vi "Read Register.vi"(6 "Read Delay ms (5)":u32=5, 7 "SPI Peripheral":refnum<class "SPI Peripheral.lvclass">, 8 "error in (no error)":errorcluster, 9 "Len":u8, 10 "Register":u8 format="%.0x") -> (0 "error out":errorcluster, 1 "Data":string)   [LabVIEW 2020, in "CTI.lvlib" / "SPI Peripheral.lvclass"]
uses:
  SPI Peripheral.lvclass
  SPI Peripheral.lvclass/SPI Peripheral.ctl
  3f2eec9a-ce11-49d3-a293-9054af33640d.vi
  Session/Session.lvclass
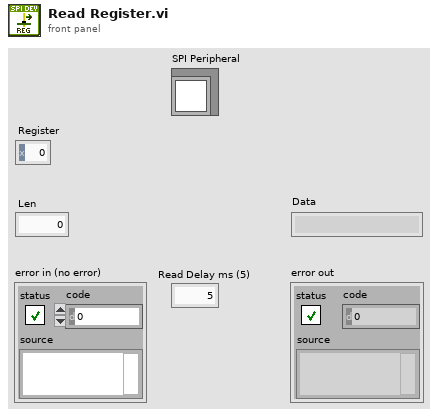
[diagram p1: front panel]
types:
  T1 = typedef "CTI.lvlib/SPI Number.ctl" = i8
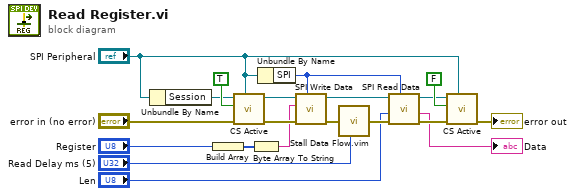
[diagram p0: block diagram]
diagram:
  n1 = Unbundle By Name("SPI Peripheral") -> ("Session"=w1:refnum<class "Session.lvclass">)
  n2 = Build Array("Register") -> (w17:u8[])
  n3 = call "CS Active.vi"("SPI Peripheral in"="SPI Peripheral", "error in (no error)"="error in (no error)", "CS Active"=TRUE, "Session In"=w1) -> ("error out"=w19:errorcluster, "Session Out"=w14:refnum<class "Session.lvclass">)  [unwired: 6 in]
  n4 = Byte Array To String(unsigned byte array=w17) -> (string=w13:string)
  n5 = Unbundle By Name("SPI Peripheral") -> ("SPI"=w8:T1)
  n6 = call "SPI Write Data.vi"("SPI #"=w8, "error in (no error)"=w19, "Data"=w13, "Session in"=w14) -> ("error out"=w15:errorcluster, "Session out"=w10:refnum<class "Session.lvclass">)  [unwired: 6 in]
  n7 = call "Stall Data Flow.vim"("value in"=w15, "milliseconds to wait"="Read Delay ms (5)") -> ("value out"=w12:errorcluster)  [unwired: 1 out]
  n8 = call "SPI Read Data.vi"("SPI #"=w8, "error in (no error)"=w12, "Len"="Len", "Session in"=w10) -> ("error out"=w5:errorcluster, "Data"=→"Data":string, "Session out"=w6:refnum<class "Session.lvclass">)  [unwired: 5 in]
  n9 = call "CS Active.vi"("SPI Peripheral in"="SPI Peripheral", "error in (no error)"=w5, "CS Active"=FALSE, "Session In"=w6) -> ("error out"=→"error out":errorcluster)  [unwired: 6 in, 1 out]
